vi "GFITS_file2fits2.vi"(10 "def_timing":string="after", 11 "file":path) -> (0 "number of before keywords":i32, 1 "before Keywords":string[][](array[string]), 2 "number of after keywords":i32, 3 "after Keywords":string[][](array[string]), 4 "all keys":string[][](array[string]), 5 "geominfo?":bool, 6 "number of total keywords":i32)   [LabVIEW 2016]
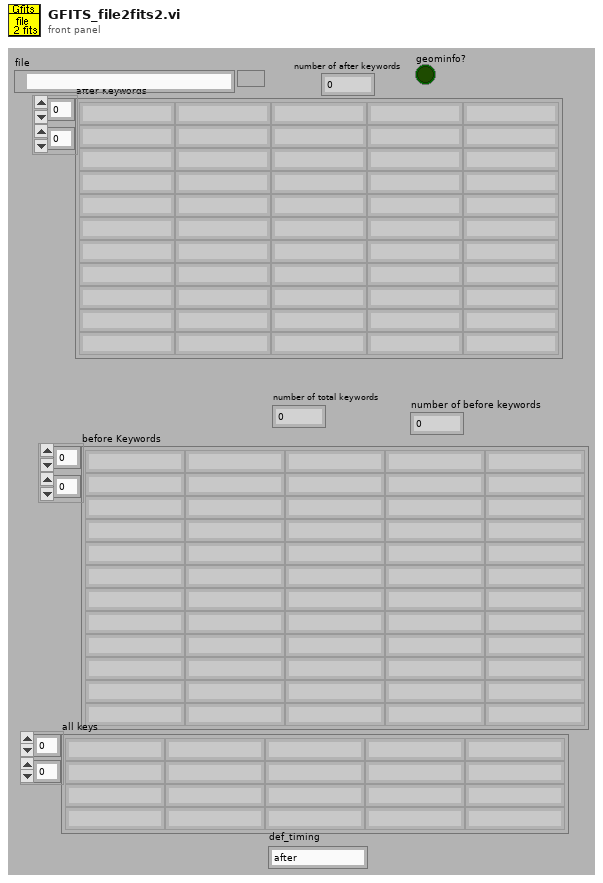
[diagram p1: front panel]
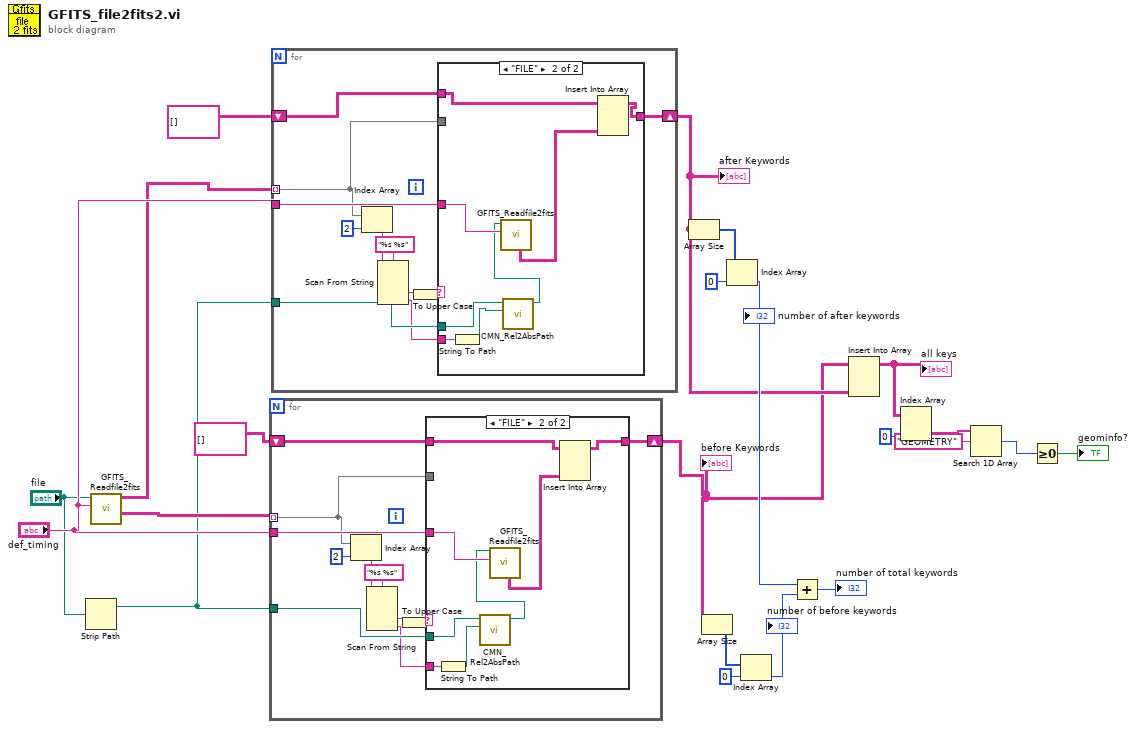
[diagram p0: block diagram]
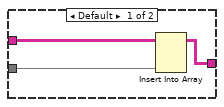
[diagram p2: hidden frame]
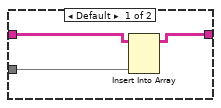
[diagram p3: hidden frame]
diagram:
  n1 = Strip Path(path="file") -> (stripped path=w17:path)  [unwired: 1 out]
  n2 = call "GFITS_Readfile2fits.vi"("def_timing"="def_timing", "file"="file") -> ("before Keywords"=w20:string[][], "after Keywords"=w19:string[][])  [unwired: 8 out]
  n3 = for {
    tunnel: w20 -> [w24] mode=indexing
    tunnel: "def_timing" -> [w28]
    tunnel: w17 -> [w27]
    shift-right: [w23] -> w1
    shift-left: string[][] [] -> [w25]
    n4 = Index Array(array=w24, index=2) -> (element=w32:string)
    n5 = Scan From String(format string="%s %s", input string=w32) -> (output 1=w30:string, output 2=w26:string)  [unwired: 2 in, 5 out]
    n6 = To Upper Case(1:w30) -> (0:w29:string)
    n7 = case shown="\"FILE\"" w29 {
      tunnel: w28 -> [_ w44]
      tunnel: w27 -> [_ w41]
      tunnel: w26 -> [_ w40]
      tunnel: w25 -> [w35 w38]
      tunnel: w24 -> [w36 _]
      tunnel: [w34 w37] -> w23
      frame Default {
        n8 = Insert Into Array(array=w35, new element=w36) -> (w34:string[][])  [unwired: 2 in]
      }
      frame "FILE" {
        n9 = String To Path(string=w40) -> (path=w43:path)
        n10 = call "CMN_Rel2AbsPath.vi"("test path"=w43, "absolute path"=w41) -> ("output path"=w42:path)  [unwired: 1 in, 8 out]
        n11 = call "GFITS_Readfile2fits.vi"("def_timing"=w44, "file"=w42) -> ("all keys"=w39:string[][])  [unwired: 9 out]
        n12 = Insert Into Array(array=w38, new element=w39) -> (w37:string[][])  [unwired: 2 in]
      }
    }
  }
  "before Keywords" <- w1
  n13 = for {
    tunnel: w19 -> [w45] mode=indexing
    tunnel: "def_timing" -> [w50]
    tunnel: w17 -> [w49]
    shift-right: [w46] -> w3
    shift-left: string[][] [] -> [w47]
    n14 = Index Array(array=w45, index=2) -> (element=w54:string)
    n15 = Scan From String(format string="%s %s", input string=w54) -> (output 1=w52:string, output 2=w48:string)  [unwired: 2 in, 5 out]
    n16 = To Upper Case(1:w52) -> (0:w51:string)
    n17 = case shown="\"FILE\"" w51 {
      tunnel: w50 -> [_ w66]
      tunnel: w49 -> [_ w64]
      tunnel: w48 -> [_ w62]
      tunnel: [w58 w59] -> w46
      tunnel: w47 -> [w57 w61]
      tunnel: w45 -> [w56 _]
      frame Default {
        n18 = Insert Into Array(array=w57, new element=w56) -> (w58:string[][])  [unwired: 2 in]
      }
      frame "FILE" {
        n19 = String To Path(string=w62) -> (path=w65:path)
        n20 = call "CMN_Rel2AbsPath.vi"("test path"=w65, "absolute path"=w64) -> ("output path"=w63:path)  [unwired: 1 in, 8 out]
        n21 = call "GFITS_Readfile2fits.vi"("def_timing"=w66, "file"=w63) -> ("all keys"=w60:string[][])  [unwired: 9 out]
        n22 = Insert Into Array(array=w61, new element=w60) -> (w59:string[][])  [unwired: 2 in]
      }
    }
  }
  "after Keywords" <- w3
  n23 = Array Size(array=w3) -> (size(s)=w13:i32[])
  n24 = Array Size(array=w1) -> (size(s)=w16:i32[])
  n25 = Index Array(array=w13, index=0) -> (element=w12:i32)
  "number of after keywords" <- w12
  n26 = Index Array(array=w16, index=0) -> (element=w11:i32)
  "number of before keywords" <- w11
  n27 = Add(x=w12, y=w11) -> (x+y=→"number of total keywords":i32)
  n28 = Insert Into Array(array=w1, new element=w3) -> (w10:string[][])  [unwired: 2 in]
  "all keys" <- w10
  n29 = Index Array(array=w10, index (col)=0 ("disabled index (col)")) -> (element=w8:string[])  [unwired: 1 in]
  n30 = Search 1D Array(1D array=w8, element="GEOMETRY") -> (index of element=w6:i32)  [unwired: 1 out]
  n31 = Greater Or Equal To 0?(x=w6) -> (x >= 0?=→"geominfo?":bool)
